vi "Create TOC Line.vi"(0 "PDF Report IN":refnum<class "PDF Report Class.lvclass">, 2 "Indentation (points)":T1=36.0, 5 "Font Ref":refnum<k24>, 7 "Font Size":T1=12.0, 9 "Width (points)":sgl, 11 "error in (no error)":errorcluster, 13 "TOC Line":T2={"Title"="", "Level"=0, "GoTo Page"=0, "GoTo Position"=0, "Destination"="", "Type & run direction"=enum."ASCII"}) -> (4 "PDF Report OUT":refnum<class "PDF Report Class.lvclass">, 8 "Paragraph":refnum<k24>, 15 "error out":errorcluster)   [LabVIEW 2019, in "Exaprom PDF.lvlib"]
doc: "Version 1.1\nDeveloped by Jean-Marc Simard\nCopyright © 2012, Exaprom Inc.\nAll rights reserved.\nLicense: BSD\n\nWith iTextSharp 4.1.6 (http://itextsharp.sourceforge.net)\nunder Mozilla Public License Version 1.1\n(http://www.mozilla.org/MPL/MPL-1.1.html)"
uses:
  LV Class/PDF Report Class/PDF Report Class.lvclass
  Controls/Chapter Controls/TOC Line.ctl
  Controls/Text Controls/Unicode/Type and run direction.ctl
  C:/work/niobrara_lv/labview pdf writer fixing/DLL/itextsharp.dll
  DLL/itextsharp.dll
  Controls/Font Controls/Font size.ctl
  Exaprom PDF.lvlib
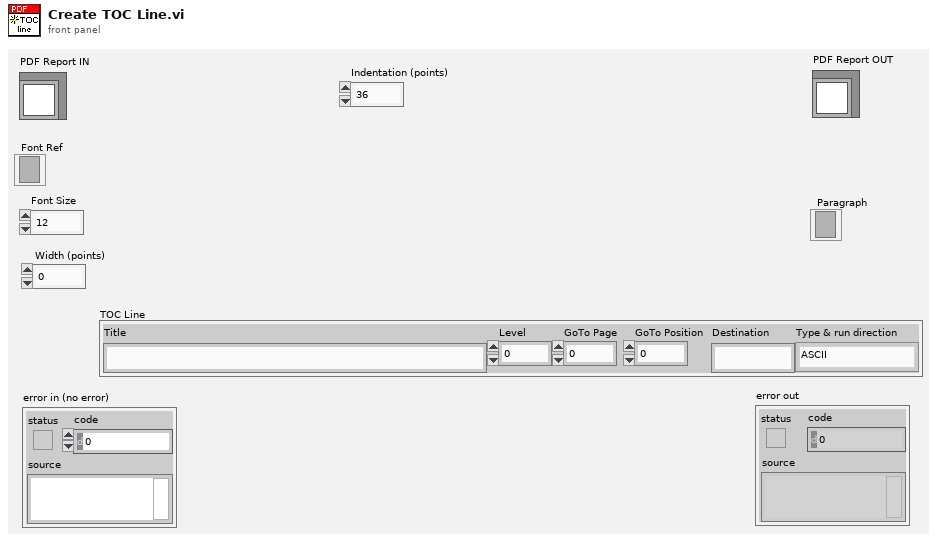
[diagram p1: front panel]
types:
  T1 = typedef "Exaprom PDF.lvlib/Font size.ctl" = sgl
  T2 = typedef "Exaprom PDF.lvlib/TOC Line.ctl" = cluster{"Title":string, "Level":u16, "GoTo Page":u16, "GoTo Position":u16, "Destination":string, "Type & run direction":T3}
  T3 = typedef "Exaprom PDF.lvlib/Type and run direction.ctl" = enum16{"Select", "ASCII", "UTF-16", "UTF-16 (default)", "UTF-16 (LTR)", "UTF-16 (RTL)"}
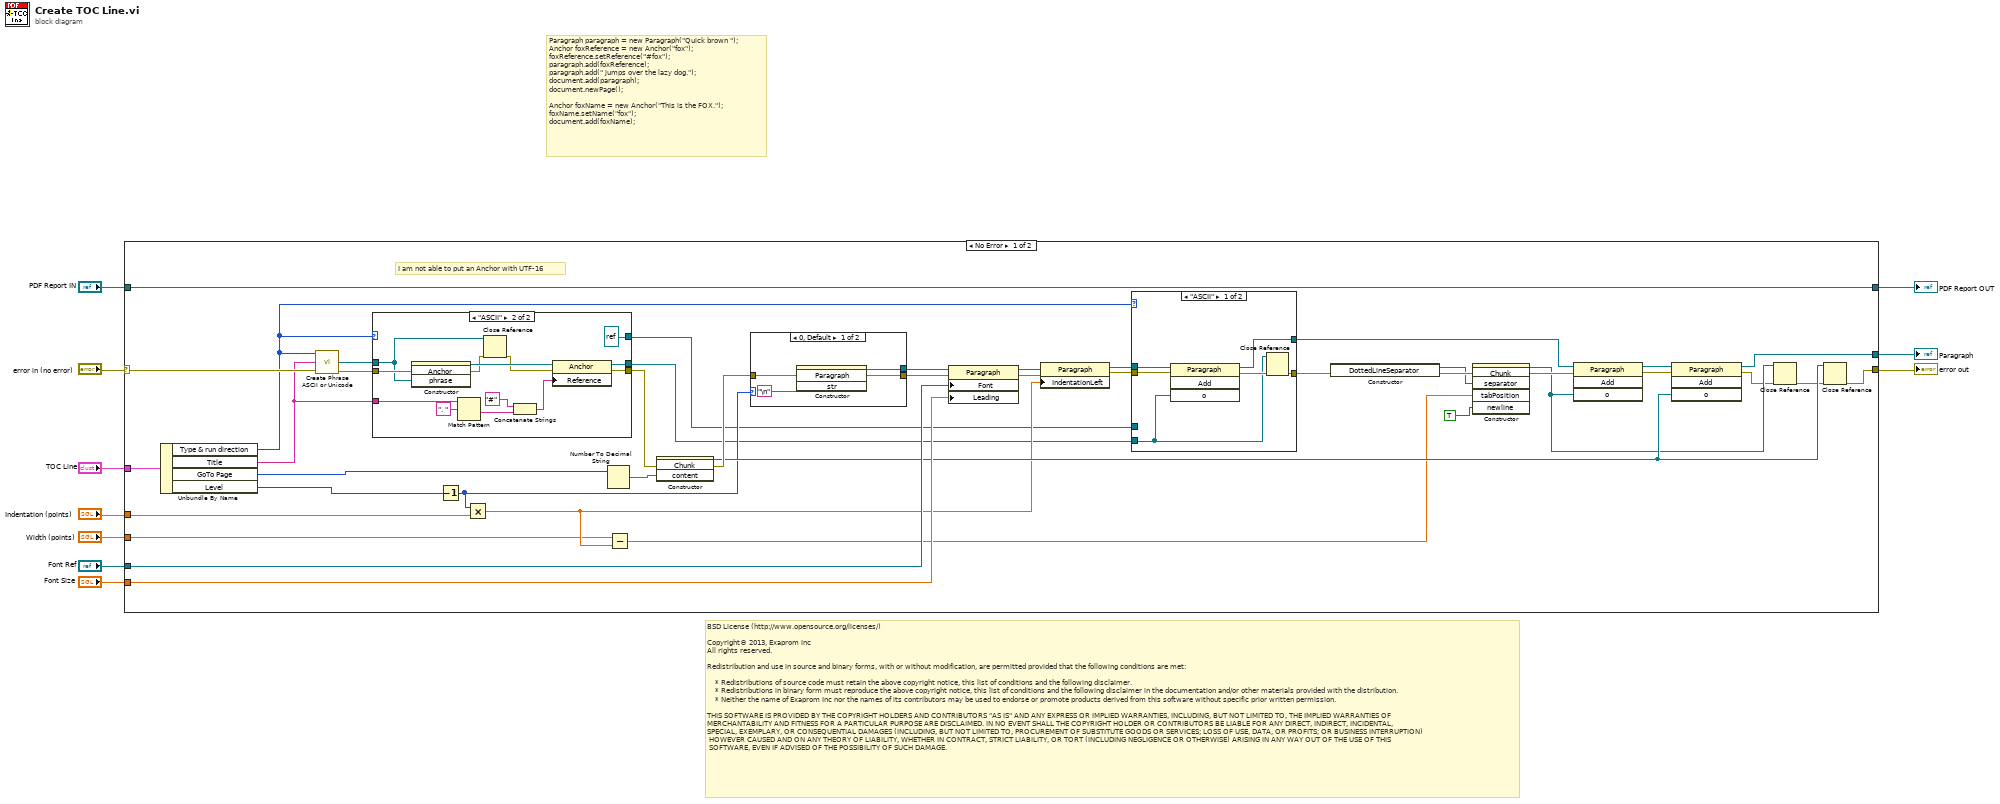
[diagram p0: block diagram]
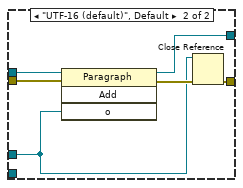
[diagram p2: hidden frame]
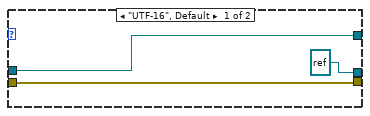
[diagram p3: hidden frame]
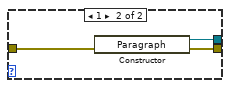
[diagram p4: hidden frame]
diagram:
  # "Paragraph paragraph = new Paragraph(\"Quick brown \");\nAnchor foxReference = new Anchor(\"fox\");\nfoxReference.setReference(\"#fox\");\nparagraph.add(foxReference);\nparagraph.add(\" jumps over the lazy dog.\");\ndocument.add(paragraph);\ndocument.newPage();\n\nAnchor foxName = new Anchor(\"This is the FOX.\");\nfoxName.setName(\"fox\");\ndocument.add(foxName);"
  # "BSD License (http://www.opensource.org/licenses/)\n\nCopyright© 2013, Exaprom Inc\nAll rights reserved.\n\nRedistribution and use in source and binary forms, with or without modification, are permitted provided that the following conditions are met:\n\n    * Redistributions of source code must retain the above copyright notice, this list of conditions and the following disclaimer.\n    * Redistributions in binary form must reproduce the above copyright notice, this list of conditions and the following disclaimer in the documentation and/or other materials provided with the distribution.\n    * Neither the name of Exaprom Inc nor the names of its contributors may be used to endorse or promote products derived from this software without specific prior written permission.\n\nTHIS SOFTWARE IS PROVIDED BY THE COPYRIGHT HOLDERS AND CONTRIBUTORS \"AS IS\" AND ANY EXPRESS OR IMPLIED WARRANTIES, INCLUDING, BUT NOT LIMITED TO, THE IMPLIED WARRANTIES OF \nMERCHANTABILITY AND FITNESS FOR A PARTICULAR PURPOSE ARE DISCLAIMED. IN NO EVENT SHALL THE COPYRIGHT HOLDER OR CONTRIBUTORS BE LIABLE FOR ANY DIRECT, INDIRECT, INCIDENTAL,\nSPECIAL, EXEMPLARY, OR CONSEQUENTIAL DAMAGES (INCLUDING, BUT NOT LIMITED TO, PROCUREMENT OF SUBSTITUTE GOODS OR SERVICES; LOSS OF USE, DATA, OR PROFITS; OR BUSINESS INTERRUPTION)\n HOWEVER CAUSED AND ON ANY THEORY OF LIABILITY, WHETHER IN CONTRACT, STRICT LIABILITY, OR TORT (INCLUDING NEGLIGENCE OR OTHERWISE) ARISING IN ANY WAY OUT OF THE USE OF THIS\n SOFTWARE, EVEN IF ADVISED OF THE POSSIBILITY OF SUCH DAMAGE."
  n1 = case shown="No Error" "error in (no error)" {
    selector: "error in (no error)" -> [w22 w87]
    tunnel: "PDF Report IN" -> [w51 w88]
    tunnel: [w51 w88] -> w9
    tunnel: [w42 w87] -> w8
    tunnel: "TOC Line" -> [w44 _]
    tunnel: "Width (points)" -> [w23 _]
    tunnel: "Font Ref" -> [w41 _]
    tunnel: "Font Size" -> [w40 _]
    tunnel: [w39 _] -> w2
    tunnel: "Indentation (points)" -> [w33 _]
    frame No Error {
      # "I am not able to put an Anchor with UTF-16"
      n2 = Unbundle By Name(w44) -> ("Type & run direction"=w12:T3, "Title"=w16:string, "GoTo Page"=w49:u16, "Level"=w34:u16)
      n3 = call "Create Phrase ASCII or Unicode.vi"("Character type"=w12, "Text"=w16, "error in (no error)"=w22) -> ("Phrase refnum"=w17:refnum<k24>, "error out"=w19:errorcluster)  [unwired: 10 in, 1 out]
      n4 = case shown="\"ASCII\"" w12 {
        tunnel: w19 -> [w66 w78]
        tunnel: [w66 w77] -> w18
        tunnel: w17 -> [w64 w73]
        tunnel: w16 -> [_ w69]
        tunnel: [refnum<k24> refnum ("new reference") w68] -> w14
        tunnel: [w64 refnum<k24> refnum ("Phrase refnum")] -> w11
        frame "UTF-16", Default {
        }
        frame "ASCII" {
          n5 = constructor class="Anchor"(error in=w78, "phrase"=w73) -> (reference out=w79:refnum<k24>, error out=w75:errorcluster)  [unwired: 2 in, 2 out]
          n6 = Match Pattern(string=w69, regular expression=". ") -> (after substring=w70:string)  [unwired: 1 in, 3 out]
          n7 = Close Reference(reference=w73, error in (no error)=w75) -> (error out=w74:errorcluster)
          n8 = Concatenate Strings("#" ("string"), w70) -> (w72:string)
          n9 = property class="Anchor"(reference=w79, error in=w74, "Reference"=w72) -> (reference out=w68:refnum<k24>, error out=w77:errorcluster)
        }
      }
      n10 = Decrement(x=w34) -> (x-1=w21:u16)
      n11 = Multiply(x=w21, y=w33) -> (x*y=w27:T1)
      n12 = Number To Decimal String(number=w49) -> (decimal integer string=w48:string)  [unwired: 1 in]
      n13 = Subtract(x=w23, y=w27) -> (x-y=w26:T1)
      n14 = constructor class="Chunk"(error in=w18, "content"=w48) -> (reference out=w32:refnum<k24>, error out=w43:errorcluster)  [unwired: 2 in, 2 out]
      n15 = case shown="0, Default" w21 {
        tunnel: [w81 w86] -> w50
        tunnel: w43 -> [w83 w85]
        tunnel: [w82 w84] -> w25
        frame 0, Default {
          n16 = constructor class="Paragraph"(error in=w83, "str"="\n") -> (reference out=w81:refnum<k24>, error out=w82:errorcluster)  [unwired: 2 in, 2 out]
        }
        frame 1 {
          n17 = constructor class="Paragraph"(error in=w85) -> (reference out=w86:refnum<k24>, error out=w84:errorcluster)  [unwired: 2 in, 1 out]
        }
      }
      n18 = property class="Paragraph"(reference=w50, error in=w25, "Font"=w41, "Leading"=w40) -> (reference out=w38:refnum<k24>, error out=w37:errorcluster)
      n19 = property class="Paragraph"(reference=w38, error in=w37, "IndentationLeft"=w27) -> (reference out=w35:refnum<k24>, error out=w36:errorcluster)
      n20 = case shown="\"ASCII\"" w12 {
        tunnel: [w57 w63] -> w47
        tunnel: w36 -> [w56 w62]
        tunnel: w35 -> [w55 w61]
        tunnel: [w53 w59] -> w15
        tunnel: w14 -> [w52 _]
        tunnel: w11 -> [_ w58]
        frame "ASCII" {
          n21 = invoke class="Paragraph" method="Add"(reference=w55, error in=w56, "o"=w52) -> (reference out=w57:refnum<k24>, error out=w54:errorcluster)  [unwired: 1 in, 2 out]
          n22 = Close Reference(reference=w52, error in (no error)=w54) -> (error out=w53:errorcluster)
        }
        frame "UTF-16 (default)", Default {
          n23 = invoke class="Paragraph" method="Add"(reference=w61, error in=w62, "o"=w58) -> (reference out=w63:refnum<k24>, error out=w60:errorcluster)  [unwired: 1 in, 2 out]
          n24 = Close Reference(reference=w58, error in (no error)=w60) -> (error out=w59:errorcluster)
        }
      }
      n25 = constructor class="DottedLineSeparator"(error in=w15) -> (reference out=w30:refnum<k24>, error out=w31:errorcluster)  [unwired: 2 in, 1 out]
      n26 = constructor class="Chunk"(error in=w31, "separator"=w30, "tabPosition"=w26, "newline"=TRUE) -> (reference out=w20:refnum<k24>, error out=w28:errorcluster)  [unwired: 2 in, 4 out]
      n27 = invoke class="Paragraph" method="Add"(reference=w47, error in=w28, "o"=w20) -> (reference out=w46:refnum<k24>, error out=w45:errorcluster)  [unwired: 1 in, 2 out]
      n28 = invoke class="Paragraph" method="Add"(reference=w46, error in=w45, "o"=w32) -> (reference out=w39:refnum<k24>, error out=w13:errorcluster)  [unwired: 1 in, 2 out]
      n29 = Close Reference(reference=w20, error in (no error)=w13) -> (error out=w24:errorcluster)
      n30 = Close Reference(reference=w32, error in (no error)=w24) -> (error out=w42:errorcluster)
    }
    frame Error {
    }
  }
  "PDF Report OUT" <- w9
  "error out" <- w8
  "Paragraph" <- w2
